vi "DrawLines.vi"(5 "VideoAccuracy [mm/px]":dbl format="%_6g", 6 "IsReverse?":bool=TRUE, 7 "Landmarkers Coordinates":u32[][](array[numeric])=[[0, 0, 0], [0, 0, 0], [0, 0, 0], [0, 0, 0], [0, 0, 0], [0, 0, 0], [0, 0, 0], [0, 0, 0], [0, 0, 0], [0, 0, 0], [0, 0, 0], [0, 0, 0], [0, 0, 0], [0, 0, 0], [0, 0, 0], [0, 0, 0], [0, 0, 0], [0, 0, 0], [0, 0, 0], [0, 0, 0], [0, 0, 0]], 8 "Antenna Coordinates":u32[][](array[numeric]), 9 "New Image":T1, 10 "In Image":T1) -> (3 "Out Image":T1)   [LabVIEW 2024]
uses:
  <vilib>/vision/Image Controls.llb/IMAQ Image.ctl
  <vilib>/vision/NI_Vision_Development_Module.lvlib
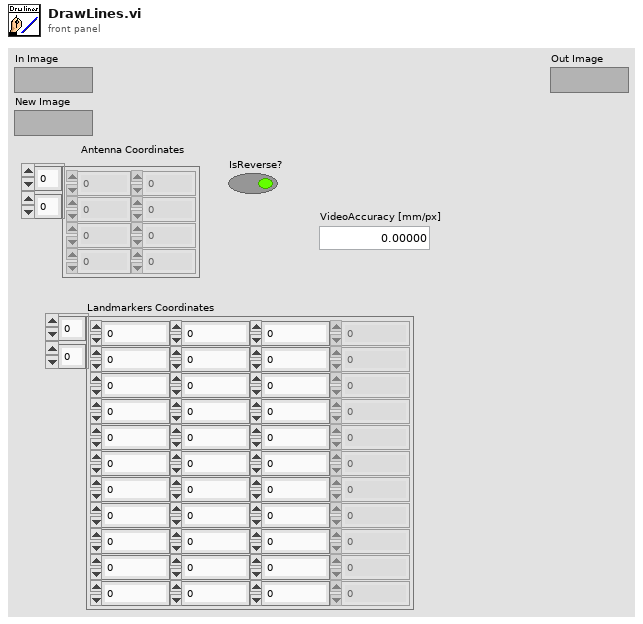
[diagram p1: front panel]
types:
  T1 = typedef "IMAQ Image.ctl" = refnum<image>
  T2 = cluster{"Desired Font (Application)":enum16{"User-specified Font", "Application Font", "System Font", "Dialog Font"}, "[User-specified Font]":cluster{"Font Name":string, "Size":i16, "Strikeout?":bool, "Italic?":bool, "Underline?":bool, "Outline?":bool, "Shadow?":bool, "Bold?":bool, "Rotation Angle":dbl}, "Horizontal Alignment":i16, "Vertical Alignment":i16}
  T3 = cluster{"Red or Hue value":u8, "Green or Sat value":u8, "Blue or Luma or Val or Inten value":u8}
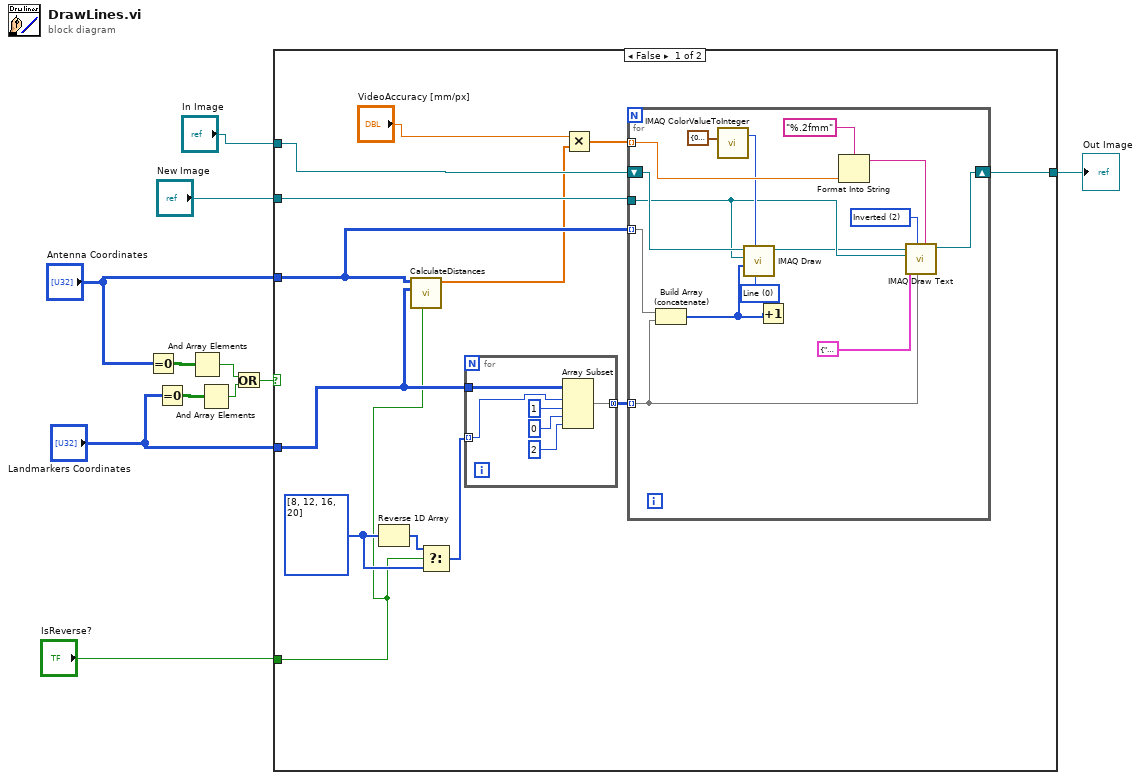
[diagram p0: block diagram]
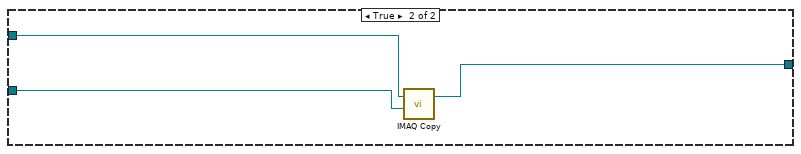
[diagram p2: hidden frame]
diagram:
  n1 = Equal To 0?(x="Antenna Coordinates") -> (x = 0?=w7:bool[][])
  n2 = Equal To 0?(x="Landmarkers Coordinates") -> (x = 0?=w6:bool[][])
  n3 = And Array Elements(Boolean array=w7) -> (logical AND=w4:bool)
  n4 = And Array Elements(Boolean array=w6) -> (logical AND=w3:bool)
  n5 = Or(x=w4, y=w3) -> (x .or. y?=w5:bool)
  n6 = case shown="False" w5 {
    tunnel: [w24 w46] -> w11
    tunnel: "New Image" -> [w23 w47]
    tunnel: "In Image" -> [w22 w48]
    tunnel: "Antenna Coordinates" -> [w17 _]
    tunnel: "Landmarkers Coordinates" -> [w16 _]
    tunnel: "IsReverse?" -> [w15 _]
    frame False {
      w19 = i32[] [8, 12, 16, 20]
      n7 = Reverse 1D Array(array=w19) -> (reversed array=w18:i32[])
      n8 = call "CalculateDistances.vi"("isReverse?"=w15, "Landmarkers Coordinates"=w16, "Antenna Coordinates"=w17) -> ("Distances"=w13:dbl[])  [unwired: 8 in]
      n9 = Select(t=w18, s=w15, f=w19) -> (s? t:f=w20:i32[])
      n10 = for {
        tunnel: w20 -> [w27] mode=indexing
        tunnel: w16 -> [w26]
        tunnel: [w25] -> w21 mode=concatenating
        n11 = Array Subset(array=w26, index (row)=w27, length (row)=1 ("length"), index (col)=0 ("index"), length (col)=2 ("length")) -> (w25:u32[][])
      }
      n12 = Multiply(x="VideoAccuracy [mm/px]", y=w13) -> (x*y=w14:dbl[])
      n13 = for {
        tunnel: w17 -> [w36] mode=indexing
        tunnel: w23 -> [w33]
        shift-right: [w38] -> w24
        shift-left: w22 -> [w44]
        tunnel: w21 -> [w37] mode=indexing
        tunnel: w14 -> [w35] mode=indexing
        w41 = 2 items=["White", "Black", "Inverted", "Black on White", "White on Black"] ("Color")
        w45 = u16 0 items=["Line", "Rectangle", "Oval"] ("Shape to draw")
        n14 = Build Array (concatenate)(w36, w37) -> (w32:u32[])
        n15 = call "IMAQ ColorValueToInteger"("Color Value"=T3 {"Red or Hue value"=0, "Green or Sat value"=0, "Blue or Luma or Val or Inten value"=255}) -> ("U32 value"=w34:u32)  [unwired: 4 in, 3 out]
        n16 = call "IMAQ Draw"("Shape to draw"=w45, "Pixel Color"=w34, "Coordinates"=w32, "Image Dst"=w33, "Image Src"=w44) -> ("Image Dst Out"=w31:T1)  [unwired: 5 in, 1 out]
        n17 = Increment(x=w32) -> ()  [unwired: 1 out]
        n18 = Format Into String(format string="%.2fmm", w35) -> (resulting string=w39:string)  [unwired: 2 in, 1 out]
        n19 = call "IMAQ Draw Text"("String"=w39, "Insertion Point"=w37, "Color"=w41, "Font, Size & Style"=T2 {"Desired Font (Application)"=enum."User-specified Font", "[User-specified Font]"={"Font Name"="", "Size"=24, "Strikeout?"=FALSE, "Italic?"=FALSE, "Underline?"=FALSE, "Outline?"=FALSE, "Shadow?"=FALSE, "Bold?"=FALSE, "Rotation Angle"=0.0}, "Horizontal Alignment"=1, "Vertical Alignment"=0}, "Image Dst"=w33, "Image Src"=w31) -> ("Image Dst Out"=w38:T1)  [unwired: 2 in, 3 out]
      }
    }
    frame True {
      n20 = call "IMAQ Copy"("Image Dst"=w47, "Image Src"=w48) -> ("Image Dst Out"=w46:T1)  [unwired: 4 in, 1 out]
    }
  }
  "Out Image" <- w11
